vi "Apply TLS options.vi"(8 "error in (no error)":errorcluster, 9 "TLS options":T1, 10 "Enable TLS?":bool, 11 "TCPSocketBasedCommHandlerBase in":refnum<class "TCPSocketBasedCommHandlerBase.lvclass">) -> (0 "error out":errorcluster, 3 "TCPSocketBasedCommHandlerBase out":refnum<class "TCPSocketBasedCommHandlerBase.lvclass">)   [LabVIEW 2020, in "wamplv.lvlib" / "TCPSocketBasedCommHandlerBase.lvclass"]
uses:
  TCPSocketBasedCommHandlerBase.lvclass
  TLS Options.ctl
  TCPSocketBasedCommHandlerBase.lvclass/TCPSocketBasedCommHandlerBase.ctl
  wamplv.lvlib
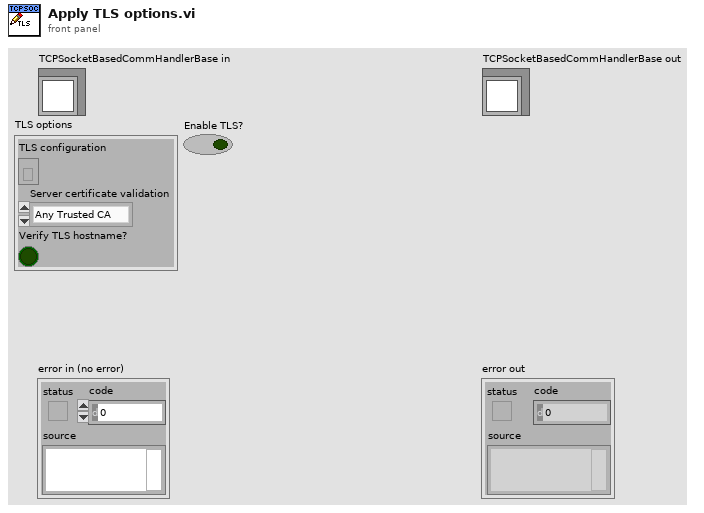
[diagram p1: front panel]
types:
  T1 = typedef "wamplv.lvlib/TLS Options.ctl" = cluster{"TLS configuration":refnum<k36>, "Server certificate validation":enum32{"Any Trusted CA", "None"}, "Verify TLS hostname?":bool}
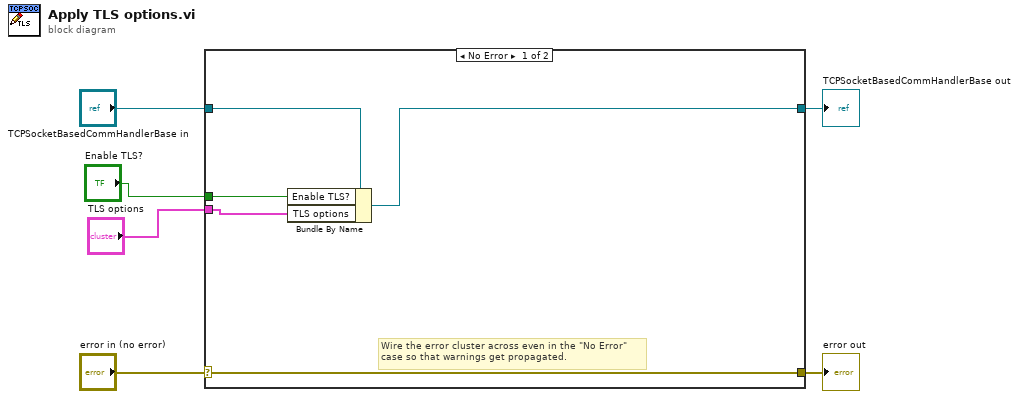
[diagram p0: block diagram]
diagram:
  n1 = case shown="No Error" "error in (no error)" {
    selector: "error in (no error)" -> [w11 w13]
    tunnel: [w11 w13] -> w5
    tunnel: [w7 w12] -> w3
    tunnel: "TCPSocketBasedCommHandlerBase in" -> [w10 w12]
    tunnel: "TLS options" -> [w9 _]
    tunnel: "Enable TLS?" -> [w8 _]
    frame No Error {
      # "Wire the error cluster across even in the \"No Error\"\ncase so that warnings get propagated."
      n2 = Bundle By Name(cluster=w10, "Enable TLS?"=w8, "TLS options"=w9) -> (w7:refnum<class "TCPSocketBasedCommHandlerBase.lvclass">)
    }
    frame Error {
    }
  }
  "error out" <- w5
  "TCPSocketBasedCommHandlerBase out" <- w3
